vi "PeriodicFilter-Format Stop Filter Entrys.vi"(7 "Seconds Since 1Jan1904 2":timestamp, 10 "Time Format String":string="%<%H:%M:%S%3u>T", 11 "Removed Info":T1[](array[typedef])) -> (3 "Array":string[](array[string]))   [LabVIEW 2017, in "Communicable State Machine.lvlib"]
uses:
  Communicable State Machine.lvlib
  Periodic String Filter Info.ctl
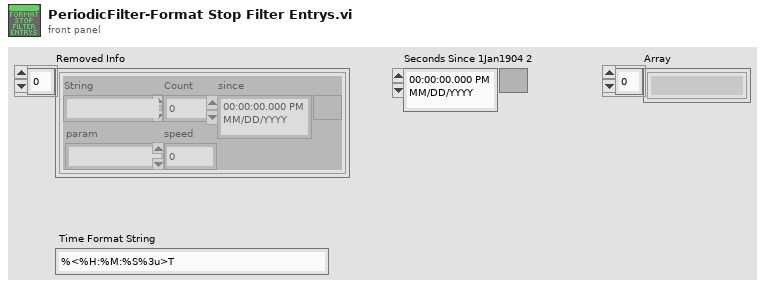
[diagram p1: front panel]
types:
  T1 = typedef "Communicable State Machine.lvlib/Periodic String Filter Info.ctl" = cluster{"String":string, "Count":i64, "since":timestamp, "param":string, "speed":dbl}
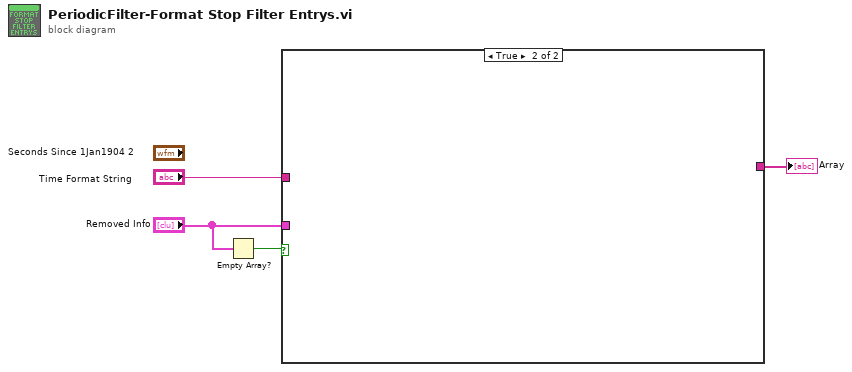
[diagram p0: block diagram]
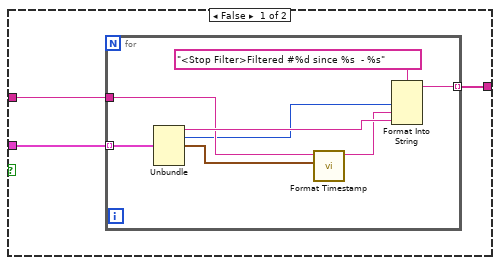
[diagram p2: hidden frame]
diagram:
  n1 = Empty Array?(array="Removed Info") -> (empty?=w1:bool)
  n2 = case shown="True" w1 {
    tunnel: "Time Format String" -> [w7 _]
    tunnel: [w6 _] -> w3
    tunnel: "Removed Info" -> [w5 _]
    frame False {
      n3 = for {
        tunnel: w5 -> [w11] mode=indexing
        tunnel: [w10] -> w6 mode=indexing
        tunnel: w7 -> [w9]
        n4 = Unbundle(w11) -> ("String"=w14:string, "Count"=w8:i64, "since"=w13:timestamp)  [unwired: 2 out]
        n5 = call "Format Timestamp.vi"("Timestamp"=w13, "Format String"=w9) -> ("String"=w12:string)  [unwired: 9 in]
        n6 = Format Into String(format string="<Stop Filter>Filtered #%d since %s  - %s", w8, w12, w14) -> (resulting string=w10:string)  [unwired: 2 in, 1 out]
      }
    }
    frame True {
    }
  }
  "Array" <- w3
